vi "BackgroundVI.vi"() -> ()   [LabVIEW 2012]
panel:
  in  "CtrlRef":refnum<vi>
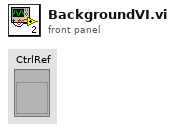
[diagram p1: front panel]
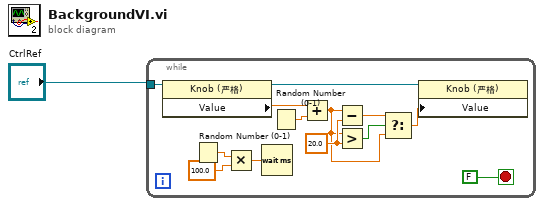
[diagram p0: block diagram]
diagram:
  n1 = while {
    tunnel: "CtrlRef" -> [w2]
    stop <- FALSE stop-if-true
    w9 = 20.0 ("y")
    n2 = property class="Knob (严格)"(reference=w2) -> (reference out=w13:refnum<vi>, "Value"=w12:dbl)  [unwired: 1 in, 1 out]
    n3 = Random Number (0-1)() -> (number: 0 to 1=w5:dbl)
    n4 = Multiply(x=w5, y=100.0) -> (x*y=w3:dbl)
    n5 = Wait (ms)(milliseconds to wait=w3) -> ()  [unwired: 1 out]
    n6 = Random Number (0-1)() -> (number: 0 to 1=w11:dbl)
    n7 = Add(x=w12, y=w11) -> (x+y=w7:dbl)
    n8 = Subtract(x=w7, y=w9) -> (x-y=w8:dbl)
    n9 = Greater?(x=w7, y=w9) -> (0:w10:bool)
    n10 = Select(t=w8, s=w10, f=w7) -> (s? t:f=w6:dbl)
    n11 = property class="Knob (严格)"(reference=w13, "Value"=w6) -> ()  [unwired: 1 in, 2 out]
  }
